vi "Reset.vi"(8 "error in (no error)":errorcluster, 11 "ChromaAcLoad in":refnum<class "ChromaAcLoad.lvclass">) -> (0 "error out":errorcluster, 3 "ChromaAcLoad out":refnum<class "ChromaAcLoad.lvclass">)   [LabVIEW 2018, in "AcPwrPlugins.lvlib" / "ChromaAcLoad.lvclass"]
doc: "This VI resets the instrument to a known state and sends initialization commands to the instrument."
uses:
  ChromaAcLoad.lvclass
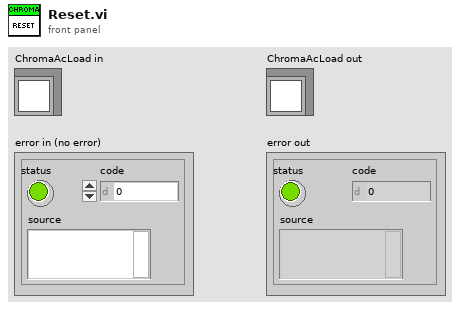
[diagram p1: front panel]
types:
  T1 = typedef "AcPwrPlugins.lvlib/ChromaAcLoad.lvclass/DeviceProperties.ctl" = cluster{"Frequency (Hz)":dbl, "Phases":cluster{"Load Resistance (Ohms)":dbl, "Load Voltage (V)":dbl, "Load Current (A)":dbl, "Load Power (W)":dbl, "Handle":string, "Name":string, "Connected":bool, "Load Current Limit (A)":dbl, "Voltage Range (V)":dbl[], "Load Current Peak (A)":dbl, "Slew Rate":cluster{"Rise Slew Rate (Units/S)":i32, "Fall Slew Rate (Units/S)":i32}, "Load Short Circuited":bool, "Line Synchronization":bool, "Crest Factor":dbl, "Power Factor":dbl, "Priority":enum16{"CF Only", "PF Only", "Both (CF)", "Both (PF)"}, "LC":cluster{"C (uF)":i32, "LS (uH)":i32, "RS (Ohm)":dbl, "RL (Ohm)":dbl}, "Timing":cluster{"TimingOn":enum16{""}, "Hours":u32, "Minutes":u32, "Seconds":dbl, "CutoffVoltage":dbl}}[], "Frequency Range(Hz)":dbl[], "Configuration Mode":enum16{"Rectified Mode (DC)", "Constant Power (DC)", "Constant Voltage (DC)", "Constant Resistance (DC)", "Constant Current (DC)", "Inrush (AC)", "RLCP (AC)", "RLC (AC)", "Constant Power (AC)", "Constant Resistance (AC)", "Constant Current (AC)"}}[]
  T2 = cluster{"Load Resistance (Ohms)":dbl, "Load Voltage (V)":dbl, "Load Current (A)":dbl, "Load Power (W)":dbl, "Handle":string, "Name":string, "Connected":bool, "Load Current Limit (A)":dbl, "Voltage Range (V)":dbl[], "Load Current Peak (A)":dbl, "Slew Rate":cluster{"Rise Slew Rate (Units/S)":i32, "Fall Slew Rate (Units/S)":i32}, "Load Short Circuited":bool, "Line Synchronization":bool, "Crest Factor":dbl, "Power Factor":dbl, "Priority":enum16{"CF Only", "PF Only", "Both (CF)", "Both (PF)"}, "LC":cluster{"C (uF)":i32, "LS (uH)":i32, "RS (Ohm)":dbl, "RL (Ohm)":dbl}, "Timing":cluster{"TimingOn":enum16{""}, "Hours":u32, "Minutes":u32, "Seconds":dbl, "CutoffVoltage":dbl}}[]
  T3 = cluster{"Load Resistance (Ohms)":dbl, "Load Voltage (V)":dbl, "Load Current (A)":dbl, "Load Power (W)":dbl, "Handle":string, "Name":string, "Connected":bool, "Load Current Limit (A)":dbl, "Voltage Range (V)":dbl[], "Load Current Peak (A)":dbl, "Slew Rate":cluster{"Rise Slew Rate (Units/S)":i32, "Fall Slew Rate (Units/S)":i32}, "Load Short Circuited":bool, "Line Synchronization":bool, "Crest Factor":dbl, "Power Factor":dbl, "Priority":enum16{"CF Only", "PF Only", "Both (CF)", "Both (PF)"}, "LC":cluster{"C (uF)":i32, "LS (uH)":i32, "RS (Ohm)":dbl, "RL (Ohm)":dbl}, "Timing":cluster{"TimingOn":enum16{""}, "Hours":u32, "Minutes":u32, "Seconds":dbl, "CutoffVoltage":dbl}}
  T4 = cluster{"Frequency (Hz)":dbl, "Phases":cluster{"Load Resistance (Ohms)":dbl, "Load Voltage (V)":dbl, "Load Current (A)":dbl, "Load Power (W)":dbl, "Handle":string, "Name":string, "Connected":bool, "Load Current Limit (A)":dbl, "Voltage Range (V)":dbl[], "Load Current Peak (A)":dbl, "Slew Rate":cluster{"Rise Slew Rate (Units/S)":i32, "Fall Slew Rate (Units/S)":i32}, "Load Short Circuited":bool, "Line Synchronization":bool, "Crest Factor":dbl, "Power Factor":dbl, "Priority":enum16{"CF Only", "PF Only", "Both (CF)", "Both (PF)"}, "LC":cluster{"C (uF)":i32, "LS (uH)":i32, "RS (Ohm)":dbl, "RL (Ohm)":dbl}, "Timing":cluster{"TimingOn":enum16{""}, "Hours":u32, "Minutes":u32, "Seconds":dbl, "CutoffVoltage":dbl}}[], "Frequency Range(Hz)":dbl[], "Configuration Mode":enum16{"Rectified Mode (DC)", "Constant Power (DC)", "Constant Voltage (DC)", "Constant Resistance (DC)", "Constant Current (DC)", "Inrush (AC)", "RLCP (AC)", "RLC (AC)", "Constant Power (AC)", "Constant Resistance (AC)", "Constant Current (AC)"}}
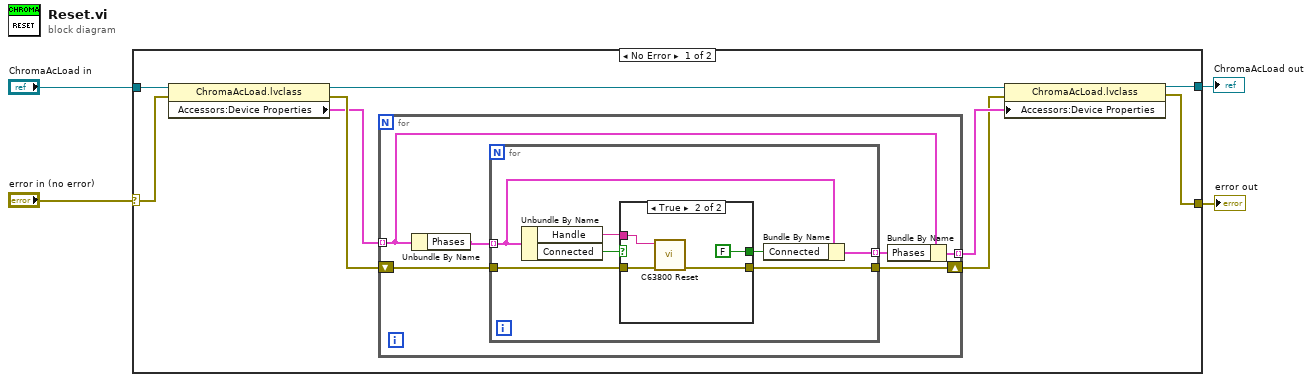
[diagram p0: block diagram]
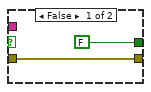
[diagram p2: hidden frame]
diagram:
  n1 = case shown="No Error" "error in (no error)" {
    selector: "error in (no error)" -> [w12 w33]
    tunnel: "ChromaAcLoad in" -> [w13 w34]
    tunnel: [w8 w34] -> w2
    tunnel: [w7 w33] -> w1
    frame No Error {
      n2 = property class="ChromaAcLoad.lvclass"(reference=w13, error in=w12) -> (reference out=w6:refnum<class "ChromaAcLoad.lvclass">, error out=w11:errorcluster, "Accessors:Device Properties"=w10:T1)
      n3 = for {
        shift-right: [w14] -> w5
        shift-left: w11 -> [w18]
        tunnel: w10 -> [w16] mode=indexing
        tunnel: [w15] -> w9 mode=indexing
        n4 = Unbundle By Name(w16) -> ("Phases"=w19:T2)
        n5 = for {
          tunnel: w19 -> [w24] mode=indexing
          tunnel: w18 -> [w26]
          tunnel: [w20] -> w17 mode=indexing
          tunnel: [w25] -> w14
          n6 = Unbundle By Name(w24) -> ("Handle"=w21:string, "Connected"=w22:bool)
          n7 = case shown="True" w22 {
            tunnel: w26 -> [w28 w29]
            tunnel: [w28 w30] -> w25
            tunnel: w21 -> [_ w31]
            tunnel: [FALSE FALSE] -> w23
            frame False {
            }
            frame True {
              n8 = call <instrlib>:"C63800 Reset.vi"("error in (no error)"=w29, "Instrument Handle"=w31) -> ("error out"=w30:errorcluster)  [unwired: 8 in, 1 out]
            }
          }
          n9 = Bundle By Name(cluster=w24, "Connected"=w23) -> (w20:T3)
        }
        n10 = Bundle By Name(cluster=w16, "Phases"=w17) -> (w15:T4)
      }
      n11 = property class="ChromaAcLoad.lvclass"(reference=w6, error in=w5, "Accessors:Device Properties"=w9) -> (reference out=w8:refnum<class "ChromaAcLoad.lvclass">, error out=w7:errorcluster)
    }
    frame Error {
    }
  }
  "error out" <- w1
  "ChromaAcLoad out" <- w2
